vi "Visa read baby.vi"() -> ()   [LabVIEW 2017]
uses:
  <vilib>/Instr/_visa.llb/VISA Configure Serial Port (Instr).vi
panel:
  out "number":u32
  out "Boolean array":bool[](array[boolean])
  out "element":bool
  out "read buffer":string
  in  "write buffer":string
  in  "VISA resource name":refnum<visa-resource-name>
  in  "Read":bool=TRUE
  out "error out":errorcluster
  out "Serial Settings:Number of Bytes at Serial Port":u32
  in  "delay":u32
  in  "Write":bool
  in  "Enable Termination\nChar (T)":bool=TRUE
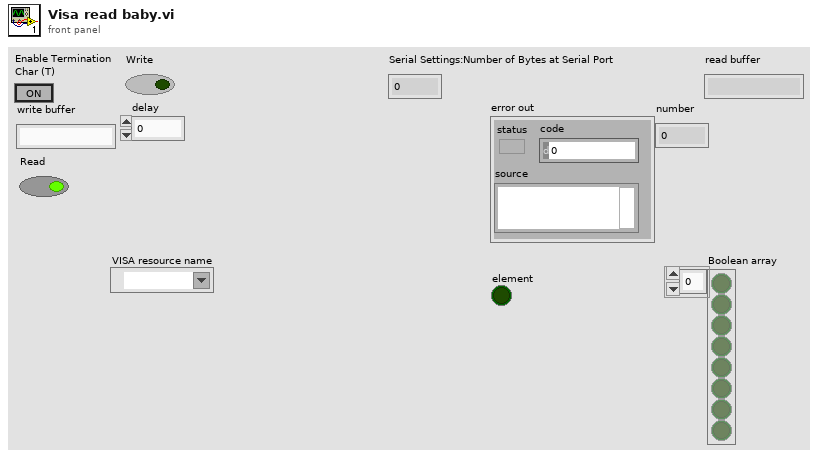
[diagram p1: front panel]
types:
  T1 = cluster{"Boolean array[0]":bool, "Boolean array[1]":bool, "Boolean array[2]":bool, "Boolean array[3]":bool, "Boolean array[4]":bool, "Boolean array[5]":bool, "Boolean array[6]":bool, "Boolean array[7]":bool}
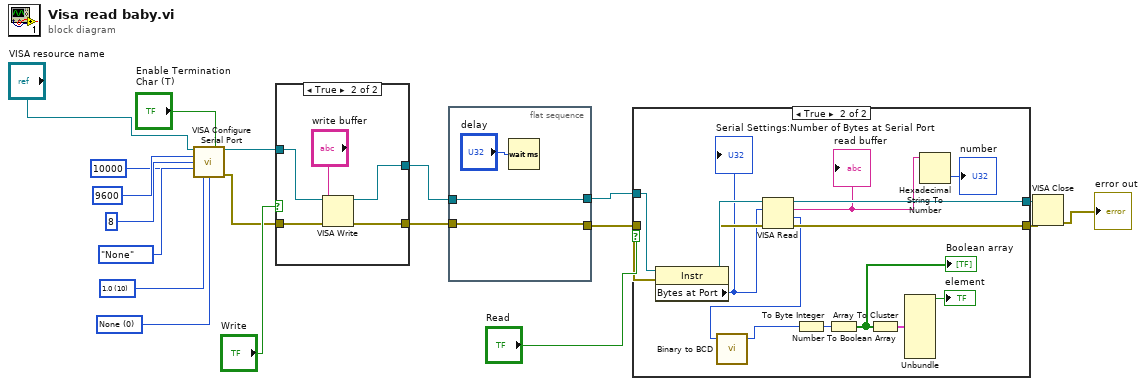
[diagram p0: block diagram]
diagram:
  w15 = u16 0 items=["None", "XON/XOFF", "RTS/CTS", "XON/XOFF & RTS/CTS", "DTR/DSR", "XON/XOFF & DTR/DSR"] ("flow control (0:none)")
  w16 = u16 10 items=["1.0"=10, "1.5"=15, "2.0"=20] ("stop bits (10: 1 bit)")
  n1 = call-poly "VISA Configure Serial Port"("VISA resource name"="VISA resource name", "timeout (10sec)"=u32 10000, "Enable Termination\nChar (T)"="Enable Termination\nChar (T)", "baud rate (9600)"=u32 9600, "data bits (8)"=u16 8, "parity (0:none)"=enum16{"None", "Odd", "Even", "Mark", "Space"}."None", "stop bits (10: 1 bit)"=w16, "flow control (0:none)"=w15) -> ("VISA resource name out"=w11:refnum<visa-resource-name>, "error out"=w10:errorcluster)  [unwired: 6 in]
  n2 = case shown="True" "Write" {
    tunnel: w11 -> [w21 w26]
    tunnel: w10 -> [w20 w25]
    tunnel: [w20 w24] -> w8
    tunnel: [w21 w23] -> w7
    frame False {
    }
    frame True {
      n3 = VISA Write(VISA resource name=w26, write buffer="write buffer", error in (no error)=w25) -> (VISA resource name out=w23:refnum<visa-resource-name>, error out=w24:errorcluster)  [unwired: 1 out]
    }
  }
  n4 = flat-sequence {
    tunnel: [w28] -> w9
    tunnel: w8 -> [w28]
    tunnel: [w27] -> w6
    tunnel: w7 -> [w27]
    frame #0 {
      n5 = Wait (ms)(milliseconds to wait="delay") -> ()  [unwired: 1 out]
    }
  }
  n6 = case shown="True" "Read" {
    tunnel: w9 -> [w31 w44]
    tunnel: w6 -> [w30 w43]
    tunnel: [w31 w41] -> w5
    tunnel: [w30 w40] -> w4
    frame False {
    }
    frame True {
      n7 = property class="Instr"(reference=w43, error in=w44) -> (reference out=w46:refnum<visa-resource-name>, error out=w45:errorcluster, "Bytes at Port"=w42:u32)
      "Serial Settings:Number of Bytes at Serial Port" <- w42
      n8 = VISA Read(VISA resource name=w46, byte count=w42, error in (no error)=w45) -> (VISA resource name out=w40:refnum<visa-resource-name>, read buffer=w34:string, return count=w33:u32, error out=w41:errorcluster)
      "read buffer" <- w34
      n9 = call <vilib>:"Binary to BCD.vi"("Binary"=w33) -> ("BCD"=w32:u8)  [unwired: 4 in]
      n10 = To Byte Integer(number=w32) -> (8bit integer=w38:i8)
      n11 = Number To Boolean Array(number=w38) -> (Boolean array=w39:bool[])
      "Boolean array" <- w39
      n12 = Array To Cluster(array=w39) -> (cluster=w36:T1)
      n13 = Unbundle(w36) -> ("Boolean array[0]"=→"element":bool)  [unwired: 7 out]
      n14 = Hexadecimal String To Number(string=w34) -> (number=→"number":u32)  [unwired: 2 in, 1 out]
    }
  }
  n15 = VISA Close(VISA resource name=w4, error in (no error)=w5) -> (error out=→"error out":errorcluster)
